vi "controll_single.vi"(9 "开关":bool=TRUE, 10 "控制编号":u8, 11 "VISA资源名称":refnum<visa-resource-name>="COM9") -> (3 "VISA资源名称输出":refnum<visa-resource-name>)   [LabVIEW 2017]
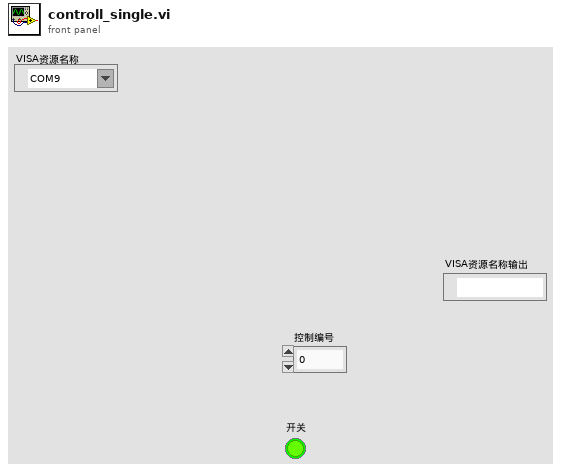
[diagram p1: front panel]
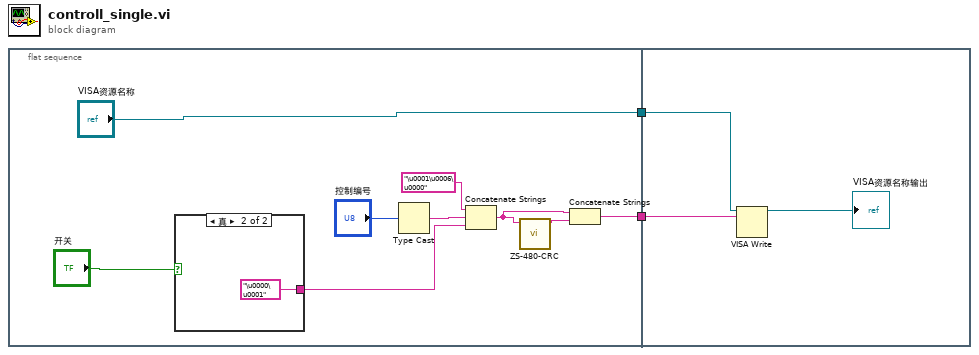
[diagram p0: block diagram]
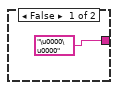
[diagram p2: hidden frame]
diagram:
  n1 = flat-sequence {
    tunnel: [w4] -> w2
    tunnel: ["VISA资源名称"] -> w1
    tunnel: w2 -> [w16]
    tunnel: w1 -> [w14]
    frame #0 {
      n2 = case shown="真" "开关" {
        tunnel: ["\u0000\u0000" ("字符串") "\u0000\u0001" ("字符串")] -> w11
        frame False {
        }
        frame True {
        }
      }
      n3 = Type Cast(x="控制编号") -> (*(type *) &x=w6:string)  [unwired: 1 in]
      n4 = Concatenate Strings("\u0001\u0006\u0000" ("字符串"), w6, w11) -> (w7:string)
      n5 = call "ZS-480-CRC.vi"("命令字符串"=w7) -> ("校验码"=w8:string)  [unwired: 10 in]
      n6 = Concatenate Strings(w7, w8) -> (w4:string)
    }
    frame #1 {
      n7 = VISA Write(VISA resource name=w14, write buffer=w16) -> (VISA resource name out=→"VISA资源名称输出":refnum<visa-resource-name>)  [unwired: 1 in, 2 out]
    }
  }
